vi "Stream Object Reference..FGV.vi"(6 "Connection Name":string, 7 "FGV State (GET)":T1, 8 "error in (no error)":errorcluster, 11 "Stream ref in":refnum<k24>) -> (0 "error out":errorcluster, 3 "Stream ref out":refnum<k24>)   [LabVIEW 2019, in "LabSSH.lvlib"]
doc: "<License>This software is distributed under the BSD 3-Clause License. For the full license please see license.txt or visit www.labvolution.com/license</License>"
uses:
  LabSSH.lvlib
  FGV State..enum.ctl
  C:/Users/modom/Dropbox/Robot/ERAA_PROJETS/HEXAP/ERAA_HEXAP_COM/ERAA_COM_HEXAP/Sous-Vi/SSH/References/Renci.SshNet.dll
  References/Renci.SshNet.dll
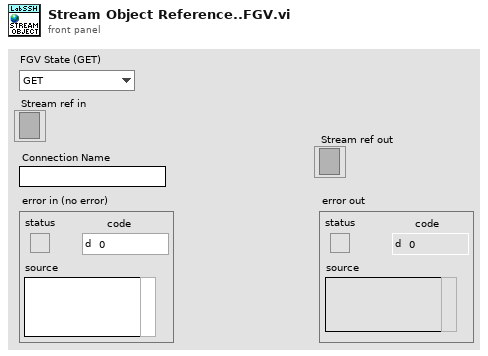
[diagram p1: front panel]
types:
  T1 = typedef "LabSSH.lvlib/FGV State..enum.ctl" = enum16{"GET", "SET"}
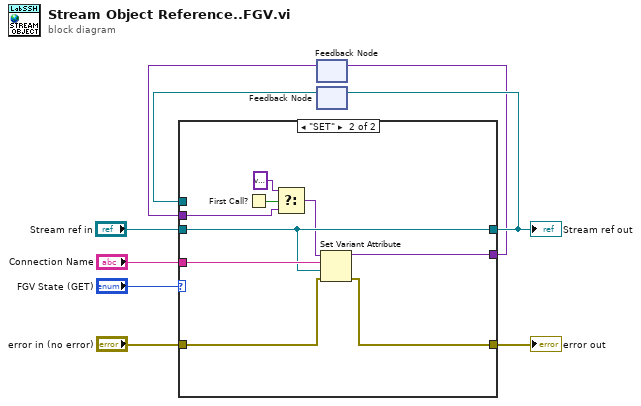
[diagram p0: block diagram]
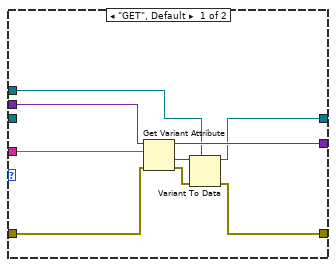
[diagram p2: hidden frame]
diagram:
  n1 = feedback #1() -> (w1:variant)  [unwired: 1 in]
  n2 = feedback #2() -> (w6:refnum<k24>)  [unwired: 1 in]
  n3 = case shown="\"SET\"" "FGV State (GET)" {
    tunnel: "error in (no error)" -> [w11 w27]
    tunnel: [w10 w26] -> w8
    tunnel: "Stream ref in" -> [_ w24]
    tunnel: [w12 w24] -> w4
    tunnel: w6 -> [w13 _]
    tunnel: "Connection Name" -> [w15 w25]
    tunnel: [w16 w23] -> w2
    tunnel: w1 -> [w14 w20]
    frame "GET", Default {
      n4 = Get Variant Attribute(Variant=w14, name=w15, error in=w11) -> (duplicate Variant=w16:variant, value=w17:variant, error out=w18:errorcluster)  [unwired: 1 in, 1 out]
      n5 = Variant To Data(error in=w18, type=w13, Variant=w17) -> (data=w12:refnum<k24>, error out=w10:errorcluster)
    }
    frame "SET" {
      n6 = First Call?() -> (First Call?: T/F=w21:bool)
      n7 = Select(t=variant ("variant"), s=w21, f=w20) -> (s? t:f=w19:variant)
      n8 = Set Variant Attribute(Variant=w19, name=w25, value=w24, error in=w27) -> (Variant out=w23:variant, error out=w26:errorcluster)  [unwired: 1 out]
    }
  }
  "error out" <- w8
  "Stream ref out" <- w4
  n9 = feedback-in #1(w2) -> ()
  n10 = feedback-in #2(w4) -> ()
